vi "PL_model.vi"(3 "output control":T1, 4 "data":variant, 5 "X":dbl[](array[numeric]), 6 "a":dbl[](array[numeric])) -> (0 "error out":errorcluster, 1 "f'(X,a)":dbl[][](array[numeric]), 2 "f(X,a)":dbl[](array[numeric]))   [LabVIEW 2014]
doc: "This template is the starting point for creating a model function to be passed to the Nonlinear Curve Fit.vi."
uses:
  <vilib>/gmath/NumericalOptimization/LM_output select.ctl
  <vilib>/gmath/NI_Gmath.lvlib
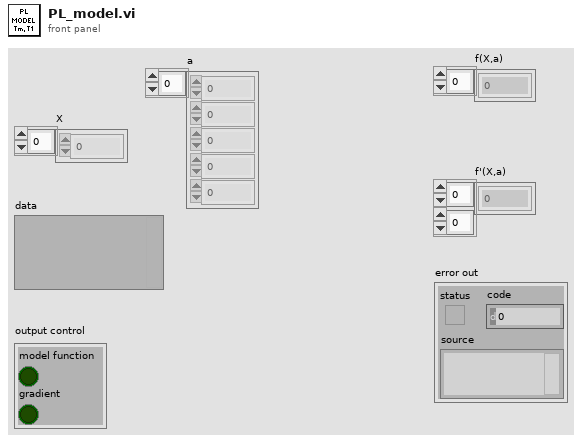
[diagram p1: front panel]
types:
  T1 = typedef "NI_Gmath.lvlib/LM_output select.ctl" = cluster{"model function":bool, "gradient":bool}
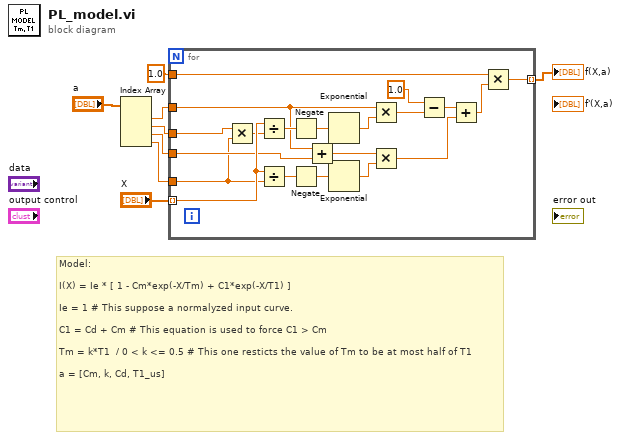
[diagram p0: block diagram]
diagram:
  # "Model:\n\nI(X) = Ie * [ 1 - Cm*exp(-X/Tm) + C1*exp(-X/T1) ]\n\nIe = 1 # This suppose a normalyzed input curve.\n\nC1 = Cd + Cm # This equation is used to force C1 > Cm\n\nTm = k*T1  / 0 < k <= 0.5 # This one resticts the value of Tm to be at most half of T1\n\na = [Cm, k, Cd, T1_us]"
  n1 = Index Array(array="a") -> (element #1=w5:dbl, element #2=w4:dbl, element #3=w3:dbl, element #4=w2:dbl)  [unwired: 4 in]
  n2 = for {
    tunnel: 1.0 ("Numeric") -> [w17]
    tunnel: w5 -> [w12]
    tunnel: w4 -> [w11]
    tunnel: w3 -> [w14]
    tunnel: w2 -> [w9]
    tunnel: [w16] -> w7 mode=indexing
    tunnel: "X" -> [w15] mode=indexing
    n3 = Multiply(x=w11, y=w9) -> (x*y=w10:dbl)
    n4 = Divide(x=w15, y=w10) -> (x/y=w28:dbl)
    n5 = Divide(x=w15, y=w9) -> (x/y=w27:dbl)
    n6 = Negate(x=w28) -> (-x=w26:dbl)
    n7 = Negate(x=w27) -> (-x=w25:dbl)
    n8 = Add(x=w12, y=w14) -> (x+y=w13:dbl)
    n9 = Exponential(1:w26) -> (0:w18:dbl)
    n10 = Exponential(1:w25) -> (0:w19:dbl)
    n11 = Multiply(x=w12, y=w18) -> (x*y=w21:dbl)
    n12 = Multiply(x=w13, y=w19) -> (x*y=w23:dbl)
    n13 = Subtract(x=1.0 ("value"), y=w21) -> (x-y=w22:dbl)
    n14 = Add(x=w22, y=w23) -> (x+y=w24:dbl)
    n15 = Multiply(x=w17, y=w24) -> (x*y=w16:dbl)
  }
  "f(X,a)" <- w7
